vi "case delete all except dbl.vi"   [LabVIEW 2013]
uses:
  <vilib>/Utility/traverseref.llb/TRef TravTarget.ctl
  tag bus/trunk/tag/Data Type.ctl
  tag bus/trunk/dictionary/create group specification.vi
  <vilib>/Utility/traverseref.llb/VI Scripting - Traverse.lvlib
  tag bus/trunk/tag/tag descriptor.lvclass
  <vilib>/Utility/VariantDataType/VariantType.lvlib
  tag bus/trunk/dictionary/data dictionary.lvclass
types:
  T1 = typedef "TRef TravTarget.ctl" = enum16{"FP", "BD", "Other"}
  T2 = typedef "tag bus.lvlib/tag descriptor.lvclass/Data Type.ctl" = enum16{"Double", "Single", "I64", "I32", "I16", "I8", "U64", "U32", "U16", "U8", "Boolean", "String", "Array of Double", "Array of Single", "Array of I64", "Array of I32", "Array of I16", "Array of I8", "Array of U64", "Array of U32", "Array of U16", "Array of U8", "Array of Boolean", "Array of String"}
  T3 = typedef "VariantType.lvlib/Type.ctl" = enum8{"Invalid Type", "Void", "I8", "I16", "I32", "I64", "U8", "U16", "U32", "U64", "Single Float", "Double Float", "Extended Float", "Single Complex", "Double Complex", "Extended Complex", "Enum U8", "Enum U16", "Enum U32", "Enum U64", "Single Float With Unit", "Double Float With Unit", "Extended Float With Unit", "Single Complex with Unit", "Double Complex with Unit", "Extended Complex with Unit", "Boolean", "String", "Path", "Picture", "Tag", "Array", "Cluster", "Variant", "LV Variant", "Waveform", "Timestamp", "Digital Waveform", "Digital Data", "ExpressData", "Refnum", "External Data", "VI", "Poly VI", "LabVIEW Class Instance", "Fixed Point"}
  T4 = typedef "VariantType.lvlib/TypedefInfo.ctl" = cluster{"Name":string, "Timestamp":u32}
  T5 = typedef "Component Runtime Interface.lvclass/Data Type.ctl" = enum16{"Double", "Single", "I64", "I32", "I16", "I8", "U64", "U32", "U16", "U8", "String", "Boolean", "Array of U8", "Array of U16", "Array of U32", "Array of U64", "Array of I64", "Array of I32", "Array of I16", "Array of I8", "Array of Double", "Array of Single", "Array of Boolean", "Array of String"}
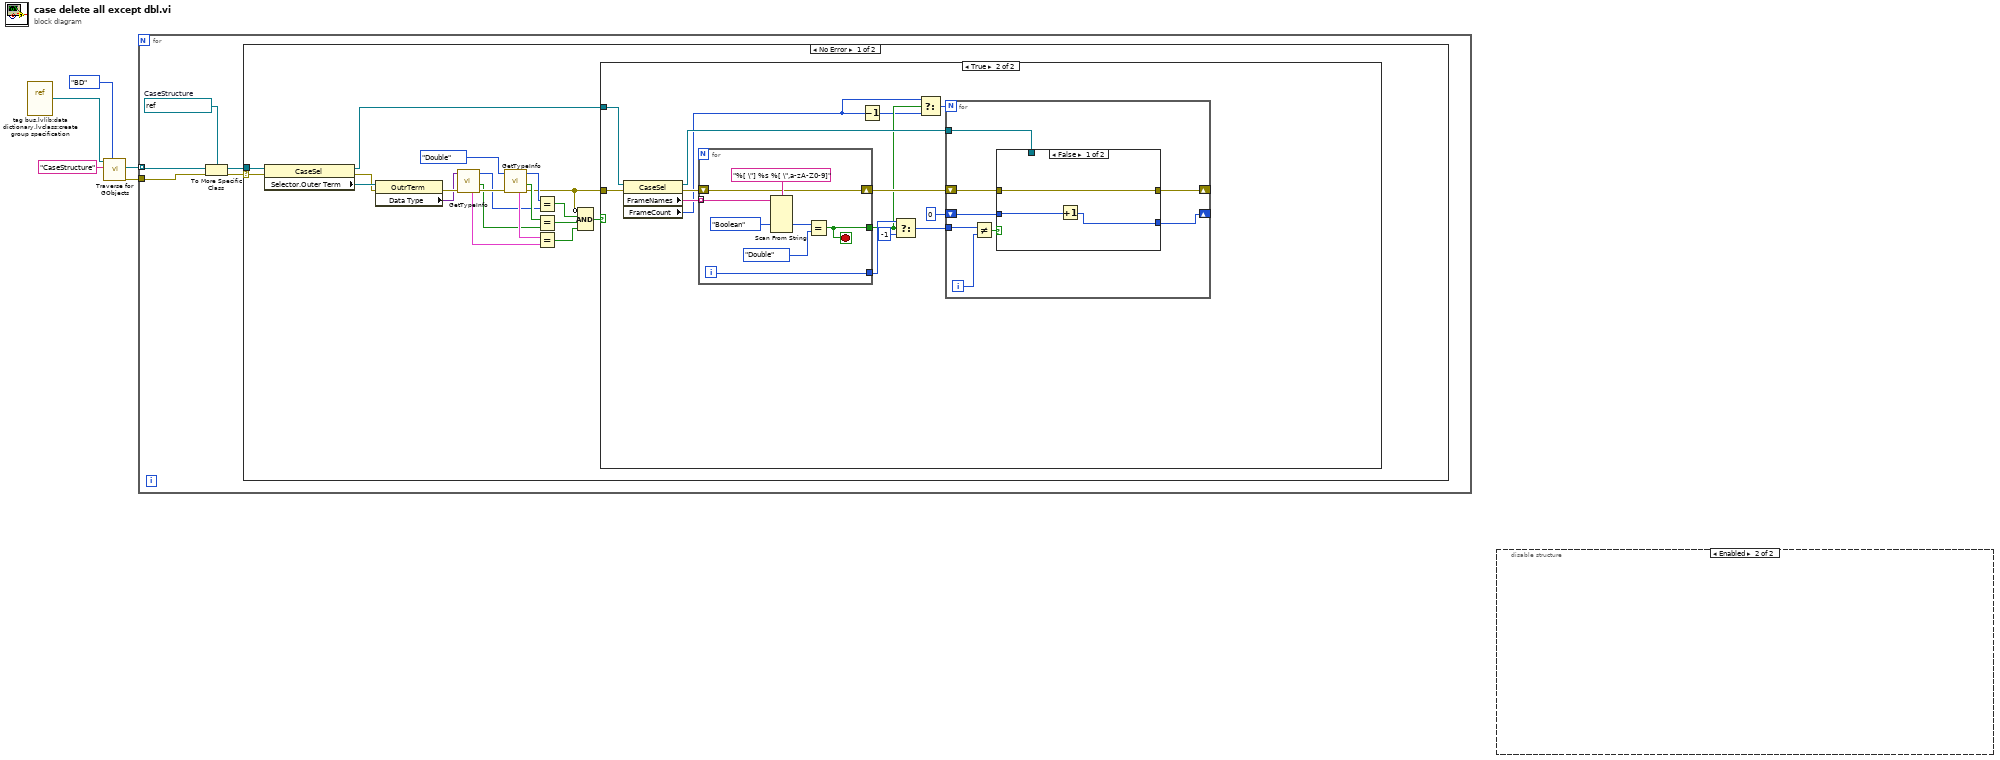
[diagram p0: block diagram]
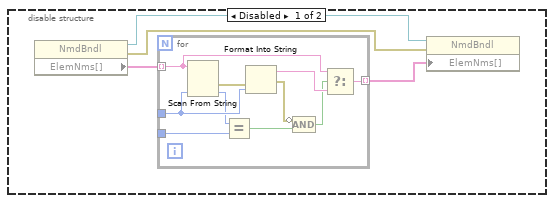
[diagram p2: hidden frame]
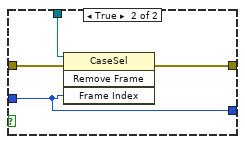
[diagram p4: hidden frame]
diagram:
  n1 = vi-ref "tag bus.lvlib:data dictionary.lvclass:create group specification.vi"() -> (w5:refnum<vi>)
  n2 = call <vilib>:"Traverse for GObjects.vi"("Traverse Target"=TRef_TravTarget."BD", "Class Name"="CaseStructure", "VI Refnum"=w5) -> ("error out"=w1:errorcluster, "References"=w2:refnum<vi>[])  [unwired: 5 in, 2 out]
  n3 = for {
    tunnel: w2 -> [w10] mode=indexing
    tunnel: w1 -> [w8]
    w9 = refnum<vi> refnum  # CaseStructure
    n4 = To More Specific Class(target class=w9, reference=w10, error in=w8) -> (specific class reference=w6:refnum<vi>, error out=w7:errorcluster)
    n5 = case shown="No Error" w7 {
      selector: w7 -> [w29 _]
      tunnel: w6 -> [w30 _]
      frame No Error {
        n6 = property class="CaseSel"(reference=w30, error in=w29) -> (reference out=w11:refnum<vi>, error out=w27:errorcluster, "Selector.Outer Term"=w28:refnum<vi>)
        n7 = property class="OutrTerm"(reference=w28, error in=w27) -> (error out=w26:errorcluster, "Data Type"=w25:variant)  [unwired: 1 out]
        n8 = call <vilib>:"GetTypeInfo.vi"("error in (no error)"=w26, "Variant"=w25) -> ("error out"=w24:errorcluster, "HasTypedef"=w16:bool, "Type Enum"=w15:T3, "TypedefInfo"=w22:T4)  [unwired: 5 in, 1 out]
        n9 = call <vilib>:"GetTypeInfo.vi"("error in (no error)"=w24, "Variant"=Data_Type."Double" ("Data Type")) -> ("error out"=w12:errorcluster, "HasTypedef"=w17:bool, "Type Enum"=w18:T3, "TypedefInfo"=w23:T4)  [unwired: 5 in, 1 out]
        n10 = Equal?(x=w18, y=w15) -> (x = y?=w19:bool)
        n11 = Equal?(x=w17, y=w16) -> (x = y?=w21:bool)
        n12 = Equal?(x=w23, y=w22) -> (x = y?=w20:bool)
        n13 = Compound Arithmetic op=AND(invert w12, w19, w21, w20) -> (w14:bool)
        n14 = case shown="True" w14 {
          tunnel: w12 -> [_ w43]
          tunnel: w11 -> [_ w44]
          frame False {
          }
          frame True {
            n15 = property class="CaseSel"(reference=w44, error in=w43) -> (reference out=w38:refnum<vi>, error out=w42:errorcluster, "FrameNames"=w41:string[], "FrameCount"=w31:i32)
            n16 = for {
              tunnel: w41 -> [w65] mode=indexing
              tunnel: [w62] -> w33
              tunnel: [w61] -> w40
              shift-right: [w60] -> w36
              shift-left: w42 -> [w60]
              i -> [w61]
              stop <- w62 stop-if-true
              n17 = Scan From String(format string="%[ \"] %s %[ \",a-zA-Z0-9]", input string=w65, default 2=Data_Type."Boolean" ("Data Type")) -> (output 2=w64:T2)  [unwired: 6 in, 3 out]
              n18 = Equal?(x=w64, y=Data_Type."Double" ("Data Type")) -> (x = y?=w62:bool)
            }
            n19 = Decrement(x=w31) -> (x-1=w32:i32)
            n20 = Select(t=w40, s=w33, f=-1) -> (s? t:f=w37:i32)
            n21 = Select(t=w31, s=w33, f=w32) -> (s? t:f=w34:i32)
            n22 = for {
              N: w34 -> [_]
              tunnel: w38 -> [w50]
              tunnel: w37 -> [w48]
              shift-right: [w51] -> _
              shift-left: w36 -> [w52]
              shift-right: [w45] -> _
              shift-left: u32 0 ("Frame Index") -> [w46]
              i -> [w47]
              n23 = Not Equal?(x=w48, y=w47) -> (x != y?=w49:bool)
              n24 = case shown="False" w49 {
                tunnel: w52 -> [w55 w59]
                tunnel: [w55 w58] -> w51
                tunnel: w50 -> [_ w57]
                tunnel: w46 -> [w54 w56]
                tunnel: [w53 w56] -> w45
                frame False {
                  n25 = Increment(x=w54) -> (x+1=w53:u32)
                }
                frame True {
                  n26 = invoke class="CaseSel" method="Remove Frame"(reference=w57, error in=w59, "Frame Index"=w56) -> (error out=w58:errorcluster)  [unwired: 1 in, 3 out]
                }
              }
            }
          }
        }
      }
      frame Error {
      }
    }
  }
  n27 = disable-structure shown="Enabled" {
    frame Disabled {
      n28 = property class="NmdBndl"() -> (reference out=w69:refnum<vi>, error out=w70:errorcluster, "ElemNms[]"=w68:string[])  [unwired: 2 in]
      n29 = for {
        tunnel: w68 -> [w81] mode=indexing
        tunnel: [w80] -> w71 mode=indexing
        tunnel: [w79] -> w72
        tunnel: [w77] -> w73
        n30 = Scan From String(input string=w81, default 1=w79) -> (error out=w83:errorcluster, output 1=w78:T5)  [unwired: 3 in, 2 out]
        n31 = Equal?(x=w78, y=w77) -> (x = y?=w76:bool)
        n32 = Format Into String(error in=w83, w79) -> (resulting string=w82:string, error out=w74:errorcluster)  [unwired: 2 in]
        n33 = Compound Arithmetic op=AND(invert w74, w76) -> (w75:bool)
        n34 = Select(t=w81, s=w75, f=w82) -> (s? t:f=w80:string)
      }
      n35 = property class="NmdBndl"(reference=w69, error in=w70, "ElemNms[]"=w71) -> ()  [unwired: 2 out]
    }
    frame Enabled {
    }
  }
